vi "cartesianToPolar.vi"(8 "Y COORDINATE":dbl, 11 "X COORDINATE":dbl) -> (0 "Hypotenuse Degrees":dbl, 3 "FEET (1)  OUTPUT":dbl)   [LabVIEW 2014]
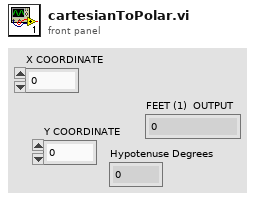
[diagram p1: front panel]
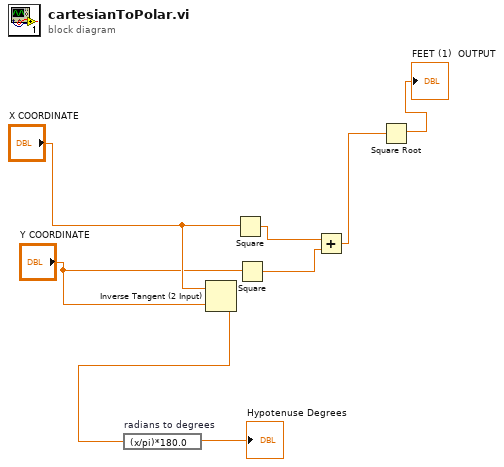
[diagram p0: block diagram]
diagram:
  n1 = Inverse Tangent (2 Input)(1:"Y COORDINATE", 2:"X COORDINATE") -> (0:w4:dbl)
  n2 = expression code="(x/pi)*180.0" "radians to degrees"(w4) -> (→"Hypotenuse Degrees":dbl)
  n3 = Square(x="X COORDINATE") -> (x^2=w7:dbl)
  n4 = Square(x="Y COORDINATE") -> (x^2=w8:dbl)
  n5 = Add(x=w7, y=w8) -> (x+y=w6:dbl)
  n6 = Square Root(x=w6) -> (sqrt(x)=→"FEET (1)  OUTPUT":dbl)
